vi "Open PCFG.vi"(8 "error in (no error)":errorcluster, 10 "Path to PCFG":path, 11 "State Cluster":T1) -> (0 "error out":errorcluster, 3 "State Cluster":T1)   [LabVIEW 2014, in "Standard Editor.lvlib"]
doc: "Open .pcfg and load into editor's system repository."
uses:
  Standard Editor.lvlib
  Controls/StateCluster.ctl
  Configuration Editor/Classes/SystemConfigRepo/SystemConfigRepo.lvclass
  Configuration Editor/Classes/Systems/Systems.lvclass
  <vilib>/NI/Configuration Framework/Node/StandardEvents.ctl
  <vilib>/NI/Configuration Framework/Node/UserEventRef.ctl
  <vilib>/NI/Configuration Framework/Controls/EventCluster.ctl
  <vilib>/NI/Configuration Framework/Node/NodeChangeEvent.ctl
  <vilib>/NI/Configuration Framework/Node/NodeRef.ctl
  <vilib>/NI/Configuration Framework/Node/NISE_CEF_Node.lvclass
  <vilib>/NI/Configuration Framework/Node/CacheState.ctl
  <vilib>/NI/Configuration Framework/Node/RefreshUIEvent.ctl
  <vilib>/NI/Configuration Framework/Node/StopEvent.ctl
  <vilib>/NI/Configuration Framework/glyph manager/glyph manager.ctl
  <vilib>/picture/picture.llb/imagedata.ctl
  <vilib>/NI/AMC/Message Queue.ctl
  <vilib>/NI/AMC/Message.ctl
  <vilib>/NI/Tools/Keyed Array/KeyedArray.ctl
  <vilib>/NI/Configuration Framework/NISE_CEF_TreeControl.lvlib
  <vilib>/NI/Configuration Framework/glyph manager/glyph manager.lvlib
  <vilib>/NI/Tools/Keyed Array/Tools_KeyedArray.lvlib
  <vilib>/NI/AMC/AMC.lvlib
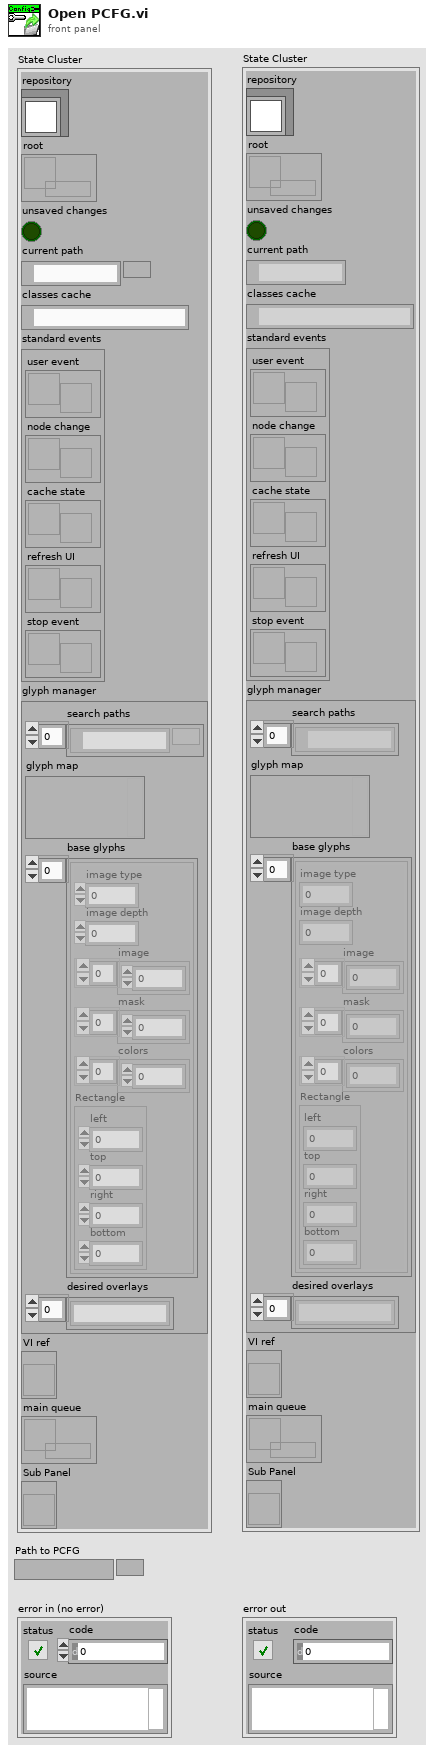
[diagram p1: front panel]
types:
  T1 = typedef "Standard Editor.lvlib/StateCluster.ctl" = cluster{"repository":refnum<class "SystemConfigRepo.lvclass">, "root":refnum<data-value>, "unsaved changes":bool, "current path":path, "classes cache":path, "standard events":T2, "glyph manager":T8, "VI ref":refnum<vi>, "main queue":T10, "Sub Panel":refnum<vi>}
  T2 = typedef "NISE_CEF_Node.lvclass/StandardEvents.ctl" = cluster{"user event":T3, "node change":T4, "cache state":T5, "refresh UI":T6, "stop event":T7}
  T3 = typedef "NISE_CEF_Node.lvclass/UserEventRef.ctl" = refnum<user-event>
  T4 = typedef "NISE_CEF_Node.lvclass/NodeChangeEvent.ctl" = refnum<user-event>
  T5 = typedef "NISE_CEF_Node.lvclass/CacheState.ctl" = refnum<user-event>
  T6 = typedef "NISE_CEF_Node.lvclass/RefreshUIEvent.ctl" = refnum<user-event>
  T7 = typedef "NISE_CEF_Node.lvclass/StopEvent.ctl" = refnum<user-event>
  T8 = typedef "glyph manager.lvlib/glyph manager.ctl" = cluster{"search paths":path[], "glyph map":variant, "base glyphs":T9[], "desired overlays":string[]}
  T9 = typedef "imagedata.ctl" = cluster{"image type":i32, "image depth":i32, "image":u8[], "mask":u8[], "colors":u32[], "Rectangle":cluster{"left":i16, "top":i16, "right":i16, "bottom":i16}}
  T10 = typedef "AMC.lvlib/Message Queue.ctl" = refnum<queue>
  T11 = typedef "NISE_CEF_Node.lvclass/NodeRef.ctl" = refnum<data-value>
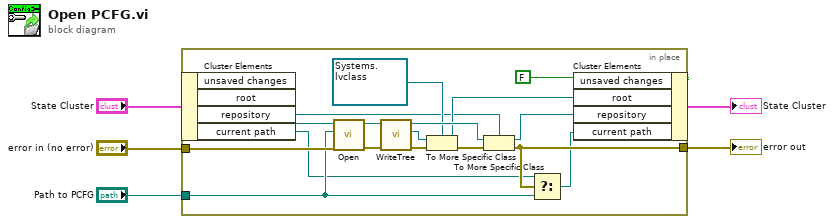
[diagram p0: block diagram]
diagram:
  n1 = in-place {
    in-place-border: "error in (no error)" -> [w21]
    in-place-border: [w14] -> w4
    in-place-border: "Path to PCFG" -> [w18]
    n2 = in-place-cluster #1("State Cluster") -> ("repository"=w9:refnum<class "SystemConfigRepo.lvclass">, "current path"=w6:path)  [unwired: 2 out]
    n3 = call-dynamic "Open.vi"("error in"=w21, "file path"=w18, "repository in"=w9) -> ("error out"=w19:errorcluster, "repository out"=w17:refnum<class "SystemConfigRepo.lvclass">)  [unwired: 6 in, 1 out]
    n4 = call-dynamic "WriteTree.vi"("error in"=w19, "repository in"=w17) -> ("error out"=w15:errorcluster, "root"=w12:T11, "repository out"=w16:refnum<class "NISE_CEF_Repository.lvclass">)  [unwired: 7 in]
    n5 = To More Specific Class(target class=refnum<data-value> refnum, reference=w12, error in=w15) -> (specific class reference=w10:refnum<data-value>, error out=w13:errorcluster)
    n6 = To More Specific Class(target class=w9, reference=w16, error in=w13) -> (specific class reference=w8:refnum<class "SystemConfigRepo.lvclass">, error out=w14:errorcluster)
    n7 = Select(t=w6, s=w14, f=w18) -> (s? t:f=w7:path)
    n8 = in-place-cluster #1("unsaved changes"=FALSE ("SaveFlag"), "root"=w10, "repository"=w8, "current path"=w7) -> (→"State Cluster":T1)
  }
  "error out" <- w4
